vi "sigError_EventCallback.vi"(4 "Error message":refnum<vi>, 5 "Event Data":T1, 6 "Control Ref":refnum<k7>, 7 "Event Common Data":T2) -> ()   [LabVIEW 2019]
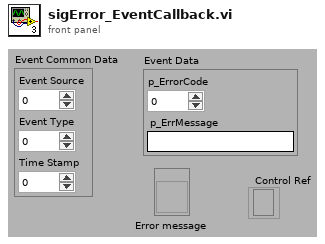
[diagram p1: front panel]
types:
  T1 = cluster{"p_ErrorCode":i32, "p_ErrMessage":string}
  T2 = cluster{"Event Source":i32, "Event Type":u32, "Time Stamp":u32}
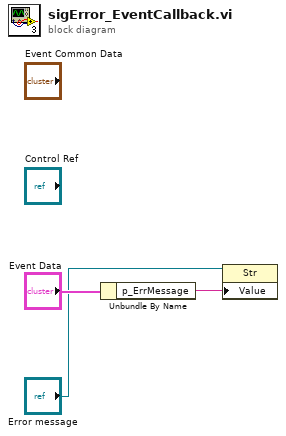
[diagram p0: block diagram]
diagram:
  n1 = Unbundle By Name("Event Data") -> ("p_ErrMessage"=w1:string)
  n2 = property class="Str"(reference="Error message", "Value"=w1) -> ()  [unwired: 1 in, 2 out]
